vi "Get All SLSC Switch Properties.vi"(8 "error in (no error)":errorcluster, 11 "SLSC Sw Custom Device Ref in":T2 format="%.0x") -> (0 "error out":errorcluster, 2 "SLSC Switch All Properties":T1, 3 "SLSC Sw Custom Device Ref out":T2 format="%.0x")   [LabVIEW 2017, in "SLSC Switch Scripting.lvlib"]
uses:
  <vilib>/NI Veristand/Custom Device API/Custom Device Item Ref.ctl
  SLSC Switch All Properties.ctl
  SLSC Switch Scripting.lvlib
  <vilib>/NI VeriStand/Custom Device API/Custom Device API.lvlib
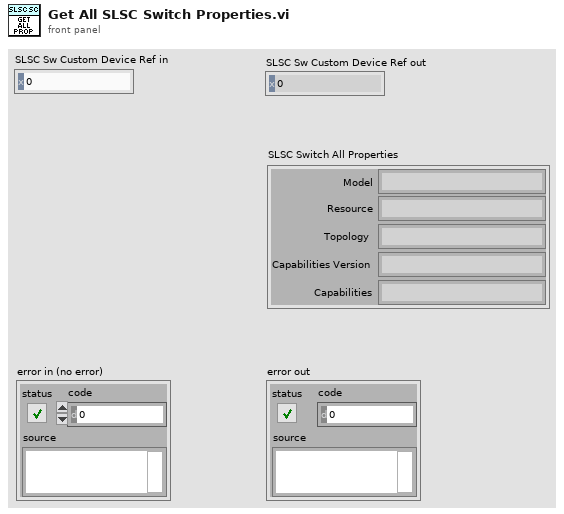
[diagram p1: front panel]
types:
  T1 = typedef "SLSC Switch Scripting.lvlib/SLSC Switch All Properties.ctl" = cluster{"Model":string, "Resource":string, "Topology":string, "Capabilities Version":string, "Capabilities":string}
  T2 = typedef "Custom Device API.lvlib/Custom Device Item Ref.ctl" = u64
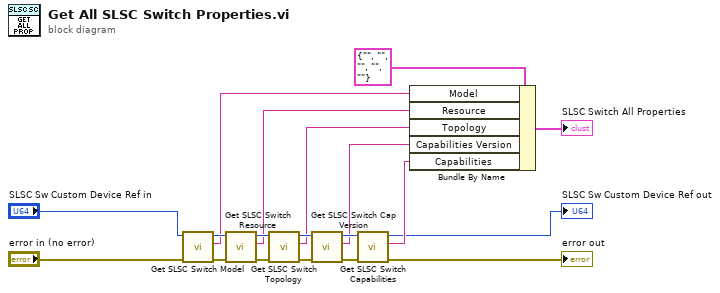
[diagram p0: block diagram]
diagram:
  n1 = call "Get SLSC Switch Model.vi"("error in (no error)"="error in (no error)", "SLSC Sw Custom Device Ref in"="SLSC Sw Custom Device Ref in") -> ("error out"=w15:errorcluster, "Model"=w7:string, "SLSC Sw Custom Device Ref out"=w13:T2)  [unwired: 7 in]
  n2 = call "Get SLSC Switch Resource.vi"("error in (no error)"=w15, "SLSC Sw Custom Device Ref in"=w13) -> ("error out"=w19:errorcluster, "Resource"=w6:string, "SLSC Sw Custom Device Ref out"=w18:T2)  [unwired: 7 in]
  n3 = call "Get SLSC Switch Topology.vi"("error in (no error)"=w19, "SLSC Sw Custom Device Ref in"=w18) -> ("error out"=w17:errorcluster, "Topology"=w5:string, "SLSC Sw Custom Device Ref out"=w16:T2)  [unwired: 7 in]
  n4 = call "Get SLSC Switch Cap Version.vi"("error in (no error)"=w17, "SLSC Sw Custom Device Ref in"=w16) -> ("error out"=w14:errorcluster, "Capabilities Version"=w4:string, "SLSC Sw Custom Device Ref out"=w11:T2)  [unwired: 7 in]
  n5 = call "Get SLSC Switch Capabilities.vi"("error in (no error)"=w14, "SLSC Sw Custom Device Ref in"=w11) -> ("error out"=→"error out":errorcluster, "Capabilities"=w3:string, "SLSC Sw Custom Device Ref out"=→"SLSC Sw Custom Device Ref out":T2)  [unwired: 7 in]
  n6 = Bundle By Name(cluster=T1 {"Model"="", "Resource"="", "Topology"="", "Capabilities Version"="", "Capabilities"=""} ("SLSC Switch All Properties"), "Model"=w7, "Resource"=w6, "Topology"=w5, "Capabilities Version"=w4, "Capabilities"=w3) -> (→"SLSC Switch All Properties":T1)
